vi "subAsyncMulti-ChannelTransceiver(NIUSRP).vi"(0 "Tx Settings":T1={"USRP IP Address"="192.168.11.4", "IQ Sampling\nRate [S/sec]"=10000000.0, "Carrier Frequency [Hz]"=87000000.0, "Start Trigger Time"={"whole seconds"=0, "fractional seconds"=0.0}, "Per Device"=[]} {"Per Device"."gain" format="%#_6f"; "Carrier Frequency [Hz]" min=50000000.0 max=6000000000.0 step=1000.0 format="%#.15p"; "IQ Sampling\nRate [S/sec]" format="%#_6p"}, 5 "Rx Settings":T1={"USRP IP Address"="192.168.11.4", "IQ Sampling\nRate [S/sec]"=10000000.0, "Carrier Frequency [Hz]"=87000000.0, "Start Trigger Time"={"whole seconds"=0, "fractional seconds"=0.0}, "Per Device"=[]} {"Per Device"."gain" format="%#_6f"; "Carrier Frequency [Hz]" min=50000000.0 max=6000000000.0 step=1000.0 format="%#.15p"; "IQ Sampling\nRate [S/sec]" format="%#_6p"}, 7 "Tx Waveforms":cdb[][](array[numeric]), 9 "apply timestamp":i32(ring) items=["Now", "Next Timebase Edge"], 11 "error in (no error)":errorcluster) -> (4 "Tx Settings (out)":T1={"USRP IP Address"="192.168.11.4", "IQ Sampling\nRate [S/sec]"=10000000.0, "Carrier Frequency [Hz]"=87000000.0, "Start Trigger Time"={"whole seconds"=0, "fractional seconds"=0.0}, "Per Device"=[]} {"Per Device"."gain" format="%#_6f"; "Carrier Frequency [Hz]" min=50000000.0 max=6000000000.0 step=1000.0 format="%#.15p"; "IQ Sampling\nRate [S/sec]" format="%#_6p"}, 6 "Rx Settings (out)":T1={"USRP IP Address"="192.168.11.4", "IQ Sampling\nRate [S/sec]"=10000000.0, "Carrier Frequency [Hz]"=87000000.0, "Start Trigger Time"={"whole seconds"=0, "fractional seconds"=0.0}, "Per Device"=[]} {"Per Device"."gain" format="%#_6f"; "Carrier Frequency [Hz]" min=50000000.0 max=6000000000.0 step=1000.0 format="%#.15p"; "IQ Sampling\nRate [S/sec]" format="%#_6p"}, 8 "Rx Waveforms":cdb[][](array[numeric]) format="%#_6p", 15 "error out":errorcluster)   [LabVIEW 2011]
uses:
  usrpHardwareSettings.ctl
  <instrlib>/niUSRP/niUSRP Timestamp.ctl
  <instrlib>/niUSRP/niUSRP Write Tx Data (2D CDB).vi
  <instrlib>/niUSRP/niUSRP Fetch Rx Data (2D CDB).vi
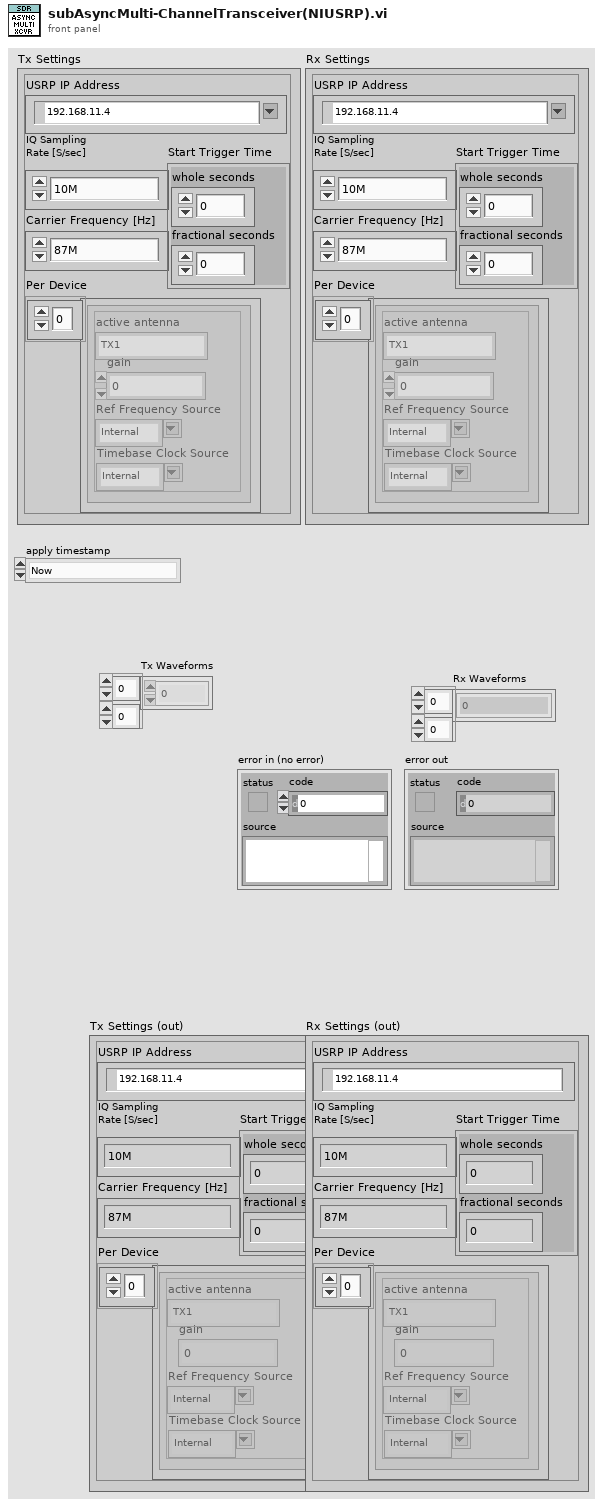
[diagram p1: front panel]
types:
  T1 = typedef "usrpHardwareSettings.ctl" = cluster{"USRP IP Address":refnum<k15>, "IQ Sampling\nRate [S/sec]":dbl, "Carrier Frequency [Hz]":dbl, "Start Trigger Time":T2, "Per Device":cluster{"active antenna":string, "gain":dbl, "Ref Frequency Source":string, "Timebase Clock Source":string}[]}
  T2 = typedef "niUSRP Timestamp.ctl" = cluster{"whole seconds":u64, "fractional seconds":dbl}
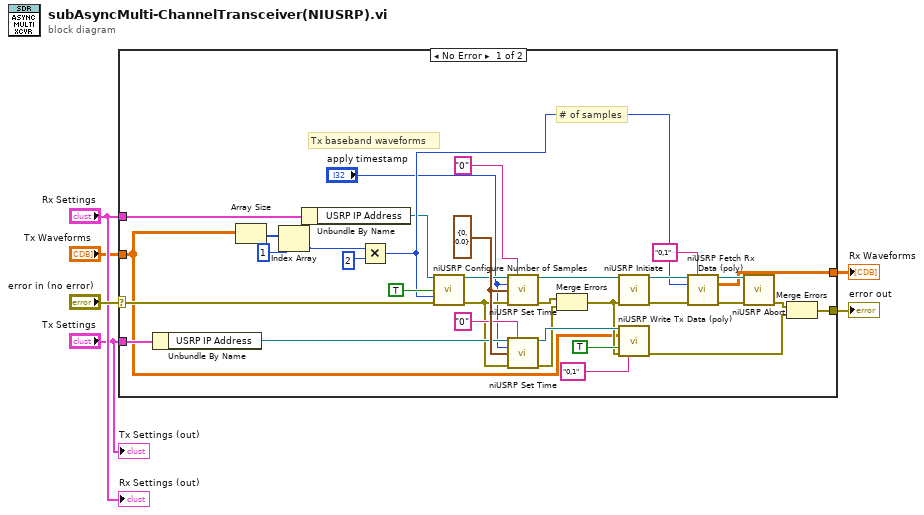
[diagram p0: block diagram]
diagram:
  n1 = case shown="No Error" "error in (no error)" {
    selector: "error in (no error)" -> [w40 w41]
    tunnel: [w18 w41] -> w5
    tunnel: "Tx Settings" -> [w33 _]
    tunnel: "Rx Settings" -> [w36 _]
    tunnel: "Tx Waveforms" -> [w8 _]
    tunnel: [w17 _] -> w1
    frame No Error {
      w38 = T2 {"whole seconds"=0, "fractional seconds"=0.0} ("timestamp")
      # "Tx baseband waveforms"
      # "# of samples"
      n2 = Unbundle By Name(w33) -> ("USRP IP Address"=w29:refnum<k15>)
      n3 = Array Size(array=w8) -> (size(s)=w12:i32[])
      n4 = Index Array(array=w12, index=1) -> (element=w11:i32)
      n5 = Unbundle By Name(w36) -> ("USRP IP Address"=w7:refnum<k15>)
      n6 = Multiply(x=w11, y=2) -> (x*y=w31:i32)
      n7 = call <instrlib>:"niUSRP Configure Number of Samples.vi"("session handle"=w7, "number of samples is finite"=TRUE, "number of samples"=w31, "error in (no error)"=w40) -> ("session handle out"=w30:refnum<k15>, "error out"=w26:errorcluster)  [unwired: 10 in]
      n8 = call <instrlib>:"niUSRP Set Time.vi"("session handle"=w30, "channel list"="0", "apply timestamp"="apply timestamp", "timestamp"=w38, "error in (no error)"=w26) -> ("session handle out"=w23:refnum<k15>, "error out"=w22:errorcluster)  [unwired: 9 in]
      n9 = call <instrlib>:"niUSRP Set Time.vi"("session handle"=w29, "channel list"="0", "apply timestamp"="apply timestamp", "timestamp"=w38, "error in (no error)"=w26) -> ("session handle out"=w25:refnum<k15>, "error out"=w24:errorcluster)  [unwired: 9 in]
      n10 = Merge Errors(w22, w24) -> (w13:errorcluster)
      n11 = call <instrlib>:"niUSRP Initiate.vi"("session handle"=w23, "error in (no error)"=w13) -> ("session handle out"=w32:refnum<k15>, "error out"=w14:errorcluster)  [unwired: 12 in]
      n12 = call-poly <instrlib>:"niUSRP Write Tx Data (poly).vi"("session handle"=w25, "channel list"="0,1", "data"=w8, "end of data?"=TRUE, "error in (no error)"=w13) -> ("error out"=w19:errorcluster)  [unwired: 9 in, 1 out]
      n13 = call-poly <instrlib>:"niUSRP Fetch Rx Data (poly).vi"("session handle"=w32, "channel list"="0,1", "number of samples"=w31, "error in (no error)"=w14) -> ("session handle out"=w37:refnum<k15>, "data"=w17:cdb[][], "error out"=w21:errorcluster)  [unwired: 8 in, 1 out]
      n14 = call <instrlib>:"niUSRP Abort.vi"("session handle"=w37, "error in (no error)"=w21) -> ("error out"=w20:errorcluster)  [unwired: 12 in, 1 out]
      n15 = Merge Errors(w20, w19) -> (w18:errorcluster)
    }
    frame Error {
    }
  }
  "error out" <- w5
  "Rx Waveforms" <- w1
  "Tx Settings (out)" <- "Tx Settings"
  "Rx Settings (out)" <- "Rx Settings"
